vi "Get Session Handle.vi"(8 "Error In":errorcluster, 11 "object in":refnum<class "AW Config.lvclass">) -> (0 "Error Out":errorcluster, 2 "Session Handle":refnum<k15>, 3 "object out":refnum<class "AW Config.lvclass">)   [LabVIEW 2023, in "AW Config.lvclass"]
uses:
  AW Config.lvclass
  AW Config.lvclass/AW Config.ctl
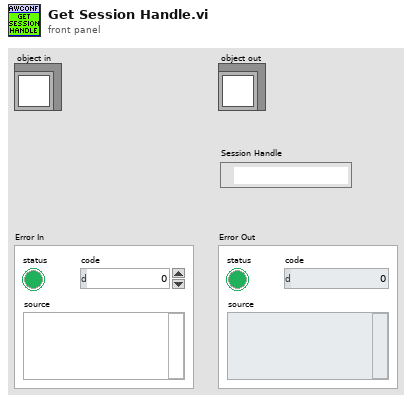
[diagram p1: front panel]
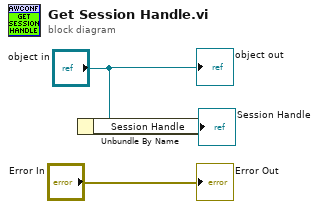
[diagram p0: block diagram]
diagram:
  n1 = Unbundle By Name("object in") -> ("Session Handle"=→"Session Handle":refnum<k15>)
  "Error Out" <- "Error In"
  "object out" <- "object in"
